vi "Cardcage Tulip Tester.vi"() -> ()   [LabVIEW 2021]
panel:
  in  "Result":string="PASS"
  in  "Test pass?":bool=TRUE
  out "Cardcage Status":string
  out "Cardcage Table":string
  out "Outset status":string
  out "Ouset Table":string
  out "Not Found?":bool
  in  "ID":string
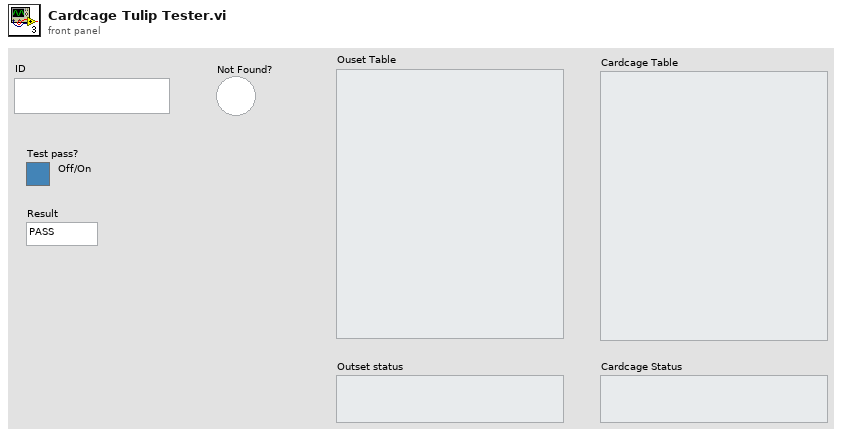
[diagram p1: front panel]
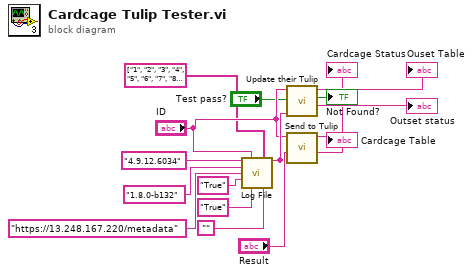
[diagram p0: block diagram]
diagram:
  n1 = call "Log File.vi"("Version"="4.9.12.6034", "ID"="ID", "Checksums"=string[] ["1", "2", "3", "4", "5", "6", "7", "8", "9", "10", "11", "12"], "Java"="1.8.0-b132", "URL"="https://13.248.167.220/metadata", "DataProcessor.exe?"="True", "Pass?"="True", "Error"="") -> ("File Name"=w13:string)  [unwired: 6 in, 1 out]
  n2 = call "Update their Tulip.vi"("Data file"=w13, "Test pass?"="Test pass?", "Serial number"="ID") -> ("Status String"=→"Outset status":string, "Not Found?"=→"Not Found?":bool, "Response body"=→"Ouset Table":string)  [unwired: 5 in, 1 out]
  n3 = call "Send to Tulip.vi"("Data file name"=w13, "Result"="Result", "Serial number"="ID") -> ("Status String"=→"Cardcage Status":string, "Response body"=→"Cardcage Table":string)  [unwired: 6 in, 1 out]
